vi "Write VIs.vi"(8 "error in (no error)":errorcluster, 10 "VIs":refnum<class "VI.lvclass">[](array[class]), 11 "Library in":refnum<class "Library.lvclass">) -> (0 "error out":errorcluster, 3 "Library out":refnum<class "Library.lvclass">)   [LabVIEW 2019]
uses:
  Library.lvclass
  VI/VI.lvclass
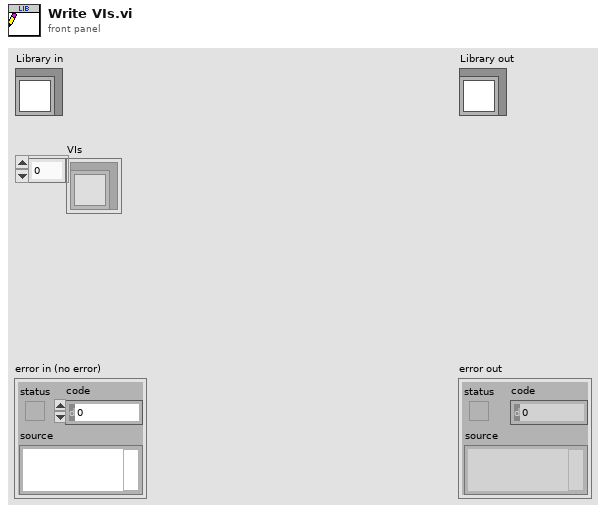
[diagram p1: front panel]
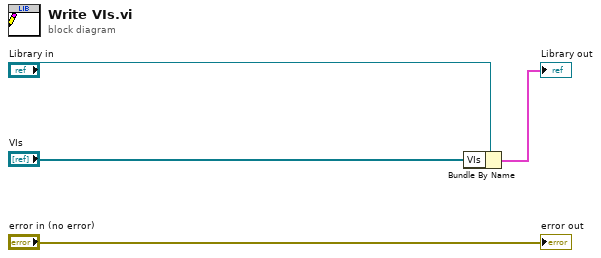
[diagram p0: block diagram]
diagram:
  n1 = Bundle By Name(cluster="Library in", "VIs"="VIs") -> (→"Library out":cluster{})
  "error out" <- "error in (no error)"
